vi "TP_Module.vi"(8 "error in":errorcluster, 11 "Queues":T1) -> (0 "error out":errorcluster)   [LabVIEW 2012]
uses:
  controls/TP_Queues.ctl
  controls/TP_Message data.ctl
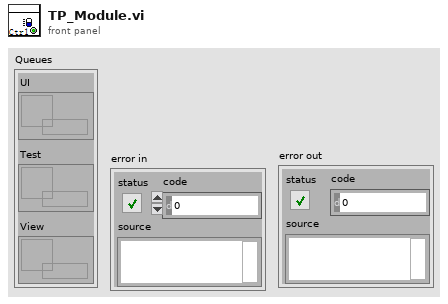
[diagram p1: front panel]
types:
  T1 = typedef "TP_Queues.ctl" = cluster{"UI":refnum<queue>, "Test":refnum<queue>, "View":refnum<queue>}
  T2 = enum16{"Init", "GetValue", "SetValue", "Destory", "ErrLog"}
  T3 = typedef "TP_Message data.ctl" = cluster{"CMD":string, "Paras":variant}
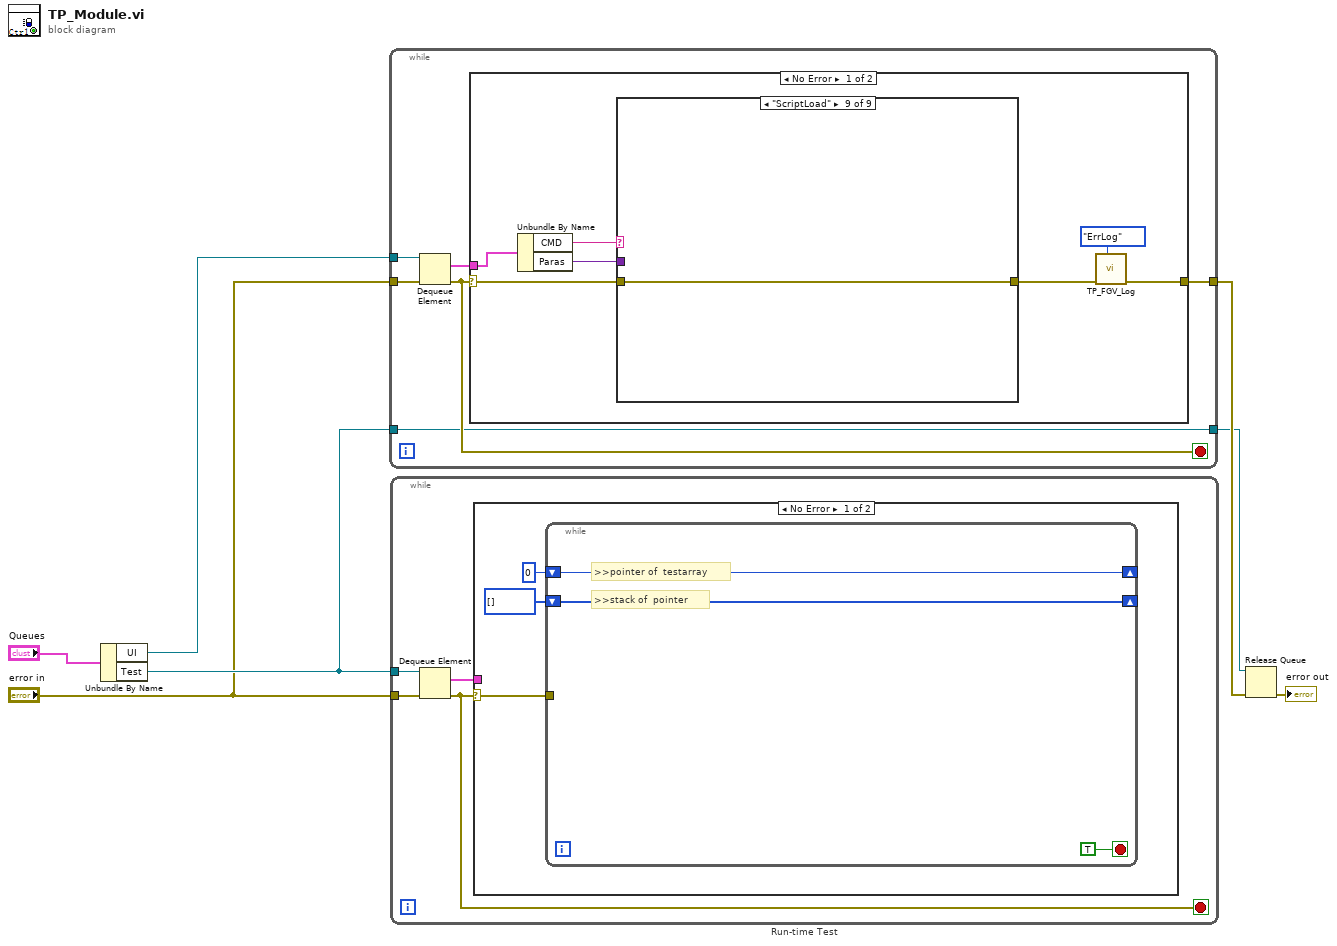
[diagram p0: block diagram]
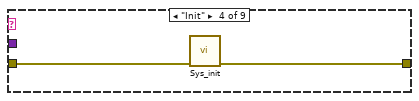
[diagram p6: hidden frame]
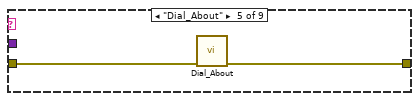
[diagram p7: hidden frame]
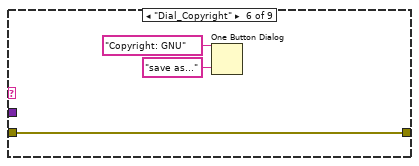
[diagram p8: hidden frame]
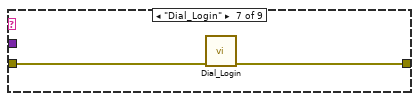
[diagram p9: hidden frame]
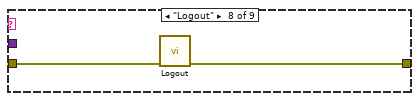
[diagram p10: hidden frame]
diagram:
  n1 = Unbundle By Name("Queues") -> ("UI"=w3:refnum<queue>, "Test"=w4:refnum<queue>)
  n2 = while {
    tunnel: w3 -> [w12]
    tunnel: "error in" -> [w13]
    tunnel: w4 -> [w8]
    tunnel: [w9] -> w7
    tunnel: [w8] -> w5
    stop <- w10 stop-if-true
    n3 = Dequeue Element(queue=w12, error in (no error)=w13) -> (element=w11:T3, error out=w10:errorcluster)  [unwired: 1 in, 2 out]
    n4 = case shown="No Error" w10 {
      selector: w10 -> [w19 w36]
      tunnel: w11 -> [w20 _]
      tunnel: [w14 w36] -> w9
      frame No Error {
        n5 = Unbundle By Name(w20) -> ("CMD"=w18:string, "Paras"=w17:variant)
        n6 = case shown="\"ScriptLoad\"" w18 {
          tunnel: w19 -> [w21 w22 w23 w25 w27 w28 w32 w34 w35]
          tunnel: w17 -> [_ _ _ _ _ _ _ _ _]
          tunnel: [w21 w22 w23 w24 w26 w28 w31 w33 w35] -> w15
          frame "Nop", Default {
          }
          frame "Exit" {
          }
          frame "Test" {
          }
          frame "Init" {
            n7 = call "Sys_init.vi"("error in"=w25) -> ("error out"=w24:errorcluster)  [unwired: 10 in]
          }
          frame "Dial_About" {
            n8 = call "Dial_About.vi"("error in"=w27) -> ("error out"=w26:errorcluster)  [unwired: 10 in]
          }
          frame "Dial_Copyright" {
            n9 = One Button Dialog(message="Copyright: GNU", button name ("OK")="save as...") -> ()  [unwired: 1 out]
          }
          frame "Dial_Login" {
            n10 = call "Dial_Login.vi"("error in"=w32) -> ("error out"=w31:errorcluster)  [unwired: 10 in]
          }
          frame "Logout" {
            n11 = call "Logout.vi"("error in (no error)"=w34) -> ("error out"=w33:errorcluster)  [unwired: 10 in]
          }
          frame "ScriptLoad" {
          }
        }
        n12 = call "TP_FGV_Log.vi"("Enum"=T2."ErrLog", "error in"=w15) -> ("error out"=w14:errorcluster)  [unwired: 9 in]
      }
      frame Error {
      }
    }
  }
  n13 = while "Run-time Test" {
    tunnel: w4 -> [w40]
    tunnel: "error in" -> [w39]
    stop <- w37 stop-if-true
    n14 = Dequeue Element(queue=w40, error in (no error)=w39) -> (element=w38:T3, error out=w37:errorcluster)  [unwired: 1 in, 2 out]
    n15 = case shown="No Error" w37 {
      selector: w37 -> [w42 _]
      tunnel: w38 -> [_ _]
      frame No Error {
        n16 = while {
          shift-right: [w46] -> _
          shift-left: 0 -> [w46]
          tunnel: w42 -> [_]
          shift-right: [w45] -> _
          shift-left: i32[] [] -> [w45]
          stop <- TRUE stop-if-true
          # ">>stack of  pointer"
          # ">>pointer of  testarray"
        }
      }
      frame Error {
      }
    }
  }
  n17 = Release Queue(queue=w5, error in (no error)=w7) -> (error out=→"error out":errorcluster)  [unwired: 1 in, 2 out]
